vi "EnQmsgs.vi"(6 "timeout in ms (-1)":i32, 7 "priority?":bool, 8 "error in (no error)":errorcluster, 9 "payload":variant, 10 "messages":string[](array[string]), 11 "EnQin":T1) -> (0 "error out":errorcluster, 3 "EnQout":T1, 4 "timed out?":bool)   [LabVIEW 2022 SP3]
uses:
  EnQref.ctl
  EnQcmd.ctl
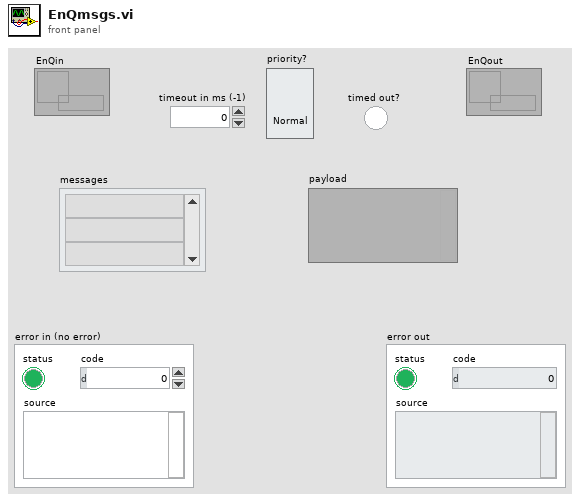
[diagram p1: front panel]
types:
  T1 = typedef "EnQref.ctl" = refnum<queue>
  T2 = typedef "EnQcmd.ctl" = cluster{"message":string, "payload":variant}
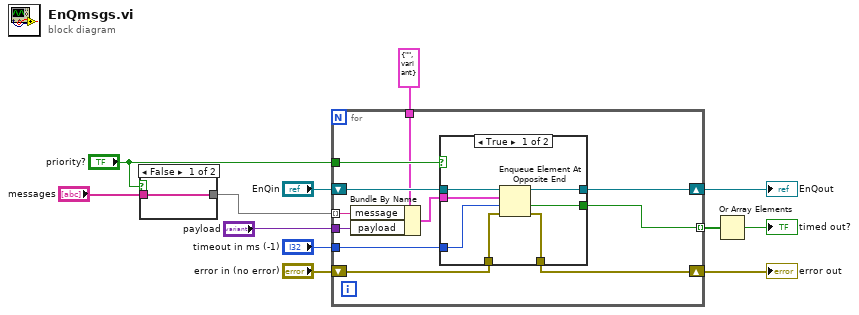
[diagram p0: block diagram]
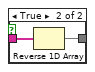
[diagram p2: hidden frame]
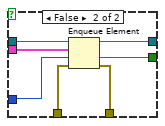
[diagram p3: hidden frame]
diagram:
  n1 = case shown="False" "priority?" {
    tunnel: "messages" -> [w13 w15]
    tunnel: [w13 w14] -> w2
    frame False {
    }
    frame True {
      n2 = Reverse 1D Array(array=w15) -> (reversed array=w14:string[])
    }
  }
  n3 = for {
    tunnel: [w22] -> w9 mode=indexing
    shift-right: [w25] -> w12
    shift-left: "EnQin" -> [w26]
    shift-right: [w23] -> w10
    shift-left: "error in (no error)" -> [w24]
    tunnel: w2 -> [w21] mode=indexing
    tunnel: "priority?" -> [w20]
    tunnel: "timeout in ms (-1)" -> [w19]
    tunnel: "payload" -> [w17]
    tunnel: T2 {"message"="", "payload"=variant} ("command") -> [w16]
    n4 = Bundle By Name(cluster=w16, "message"=w21, "payload"=w17) -> (w18:T2)
    n5 = case shown="True" w20 {
      tunnel: w26 -> [w33 w40]
      tunnel: [w32 w39] -> w25
      tunnel: w24 -> [w31 w38]
      tunnel: [w30 w37] -> w23
      tunnel: [w29 w36] -> w22
      tunnel: w18 -> [w28 w35]
      tunnel: w19 -> [w27 w34]
      frame True {
        n6 = Enqueue Element At Opposite End(queue=w33, element=w28, timeout in ms (-1)=w27, error in (no error)=w31) -> (queue out=w32:T1, timed out?=w29:bool, error out=w30:errorcluster)
      }
      frame False {
        n7 = Enqueue Element(queue=w40, element=w35, timeout in ms (-1)=w34, error in (no error)=w38) -> (queue out=w39:T1, timed out?=w36:bool, error out=w37:errorcluster)
      }
    }
  }
  "error out" <- w10
  "EnQout" <- w12
  n8 = Or Array Elements(Boolean array=w9) -> (logical OR=→"timed out?":bool)
